vi "PH_Timing.destructor.vi"(0 "i ref in":refnum<vi>, 5 "error in(no error)":errorcluster) -> (19 "error out":errorcluster)   [LabVIEW 2014, in "PH_Timing.lvlib"]
doc: "This is the destructor of a class.\n\nLicense Agreement for this software:\n\nCopyright (C)\nGesellschaft für Schwerionenforschung, GSI\nPlanckstr. 1\n64291 Darmstadt\nGermany\n\nContact: D.Beck@gsi.de \n\nThis program is free software; you can redistribute it and/or modify it under the terms of the \nGNU General Public License as published by the Free Software Foundation; either version 2 of \nthe license, or (at your option) any later version.\n\nThis program is distributed in the hope that it will be useful, but WITHOUT ANY WARRANTY; \nwithout even the implied warranty of MERCHANTABILITY or FITNESS FOR A PARTICULAR PURPOSE. See the GNU General License for more details (http://www.gnu.org).\n\nGesellschaft für Schwerionenforschung, GSI\nPlanckstr. 1, 64291 Darmstadt, Germany\nFor all questions and ideas contact: M.Richter@gsi.de, H.Brand@gsi.de or D.Beck@gsi.de.\nLast update: 16-JUN-2004"
uses:
  PH_Timing.lvlib
  lib.lib/DimLVEvent/LVDimInterface/LVDimInterface.lvlib
  PH_Switch/PH_Switch.lvlib
  CSDigitalIO/BNC555/BNC555.lvlib
  CSDigitalIO/SRDG535/SRDG535.lvlib
  PH_SRDG645/PH_SRDG645.lvlib
  PH_Common/PH_Common.lvlib
  PH_StatusHandler/PH_StatusHandler.lvlib
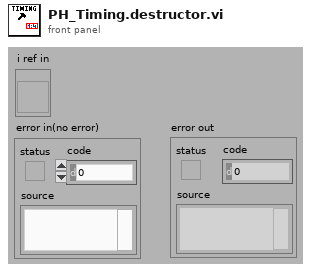
[diagram p1: front panel]
types:
  T1 = typedef "PH_Timing.lvlib/PH_Timing.i attribute.ctl" = cluster{"Sequencer":cluster{"linked?":bool, "Proc State":string, "Ref State":refnum<vi>}, "Gate Generator":cluster{"GD":cluster{"Device Status":T2, "linked?":bool}, "Settings":T3, "GUI Ref":refnum<vi>}, "Interlock Bypass":cluster{"Instancename":string, "Switch linked?":bool, "Device Status":T2, "Ref Status":refnum<vi>}, "Roughtuner":cluster{"Settings":T4, "GUI Ref":refnum<vi>, "GD":cluster{"Device Status":T2, "linked?":bool}}, "0,5Hz Gater":cluster{"Settings":T5, "GUI Ref":refnum<vi>, "GD":cluster{"Device Status":T2, "linked?":bool}}, "Slow Trigger":cluster{"Settings":T6, "GUI Ref":refnum<vi>, "Service ID Delay":i32, "Service ID Ext Trig":i32, "Wanted Settings":T6}, "Timing Mode":cluster{"Mode":T7, "GUI Ref":refnum<vi>, "Service ID T2":i32, "Service ID Mode":i32, "Wanted Mode":T7}, "ns Generator":cluster{"Settings":T8, "ns Generator Settings":refnum<vi>, "GD":cluster{"Device Status":T2, "linked?":bool}}, "Phase FEs":cluster{"Settings":T11, "GUI Ref":refnum<vi>, "Service ID Phase":i32, "Wanted Settings":T11}, "GD GUI Refs":refnum<vi>[], "Heads":T12[], "GUI Ref Delete":refnum<vi>}
  T2 = typedef "PH_StatusHandler.lvlib/PH_StatusHandler.Status.ctl" = i16
  T3 = typedef "PH_Timing.lvlib/PH_Timing.GateGen.ctl" = cluster{"Instance":string, "Channel Gate":i32, "Channel T2":i32, "Width Gate":dbl, "Width T2":dbl, "Delay Gate":dbl, "Delay T2":dbl, "Gate activ":bool, "T2 activ":bool, "System Mode":enum16{"Normal", "Single", "Burst", "Duty Cycle"}}
  T4 = typedef "PH_Timing.lvlib/PH_Timing.Roughtuner.ctl" = cluster{"Instance":string, "Phase PHELIX / UNILAC":cluster{"Channel":u16, "relative to":u16, "Delay [ms]":dbl}, "Pulse Length":cluster{"Channel":u16, "relative to":u16, "Delay [ms]":dbl}, "Trigger":cluster{"externally?":bool, "Rate [Hz]":dbl}}
  T5 = typedef "PH_Timing.lvlib/PH_Timing.0.5HzGater.ctl" = cluster{"Instance":string, "Channel ns FE Delay":i32, "Channel 0.5Hz":i32, "Width ns FE Delay":dbl, "Width 0.5Hz":dbl, "Delay ns FE Delay":dbl, "Delay 0.5Hz":dbl, "ns FE Delay active":bool, "0.5Hz activ":bool, "ns FE Delay inverted":bool, "0.5Hz inverted":bool}
  T6 = typedef "PH_Timing.lvlib/PH_Timing.Slow Trigger Settings.ctl" = cluster{"Delay":dbl, "externally triggered?":bool}
  T7 = typedef "PH_Timing.lvlib/PH_Timing.Timing Mode.ctl" = cluster{"T2":i16, "Modeselector":enum32{"10 Hz", "0.5 Hz", "Shot"}}
  T8 = typedef "PH_Timing.lvlib/PH_Timing.ns Generator.ctl" = cluster{"Instance":string, "Phase fs / ns FE":cluster{"Channel":T9, "Settings":T10}}
  T9 = typedef "Stanford Research DG645 - Driver.lvlib/Channel.ctl" = i32
  T10 = typedef "PH_SRDG645.lvlib/PH_SRDG645.Channel Settings.ctl" = cluster{"Delay [s]":dbl, "relative to":i32}
  T11 = typedef "PH_Timing.lvlib/PH_Timing.Phase FEs.ctl" = cluster{"Phase":dbl}
  T12 = typedef "PH_Timing.lvlib/PH_Timing.PU Data.ctl" = cluster{"linked?":bool, "Data":T13, "GD":cluster{"Device Status":T2, "linked?":bool}, "GUI Ref":refnum<vi>, "PU":T14}
  T13 = typedef "PH_Timing.lvlib/PH_Timing.PU Info.ctl" = cluster{"Act CH?":bool, "GD":string, "CH":i32, "Delay":dbl, "active":bool, "in Use?":bool}
  T14 = typedef "PH_PP_Common.lvlib/PH_PP_Common.PUs.ctl" = enum16{"no Info", "PA-19mm-1", "PA-19mm-2", "PA-45mm-PILC", "PA-45mm-MAIN", "MA-PU-1", "MA-PU-2", "MA-PU-3", "MA-PU-4", "MA-PU-5", "MA-PU-6", "MA-FR", "MA-PILC", "PA-45mm-DP"}
  T15 = enum16{"SetAttribute", "GetAttribute", "CreateAttribute", "DestroyAttribute", "DestroyAllAtributes"}
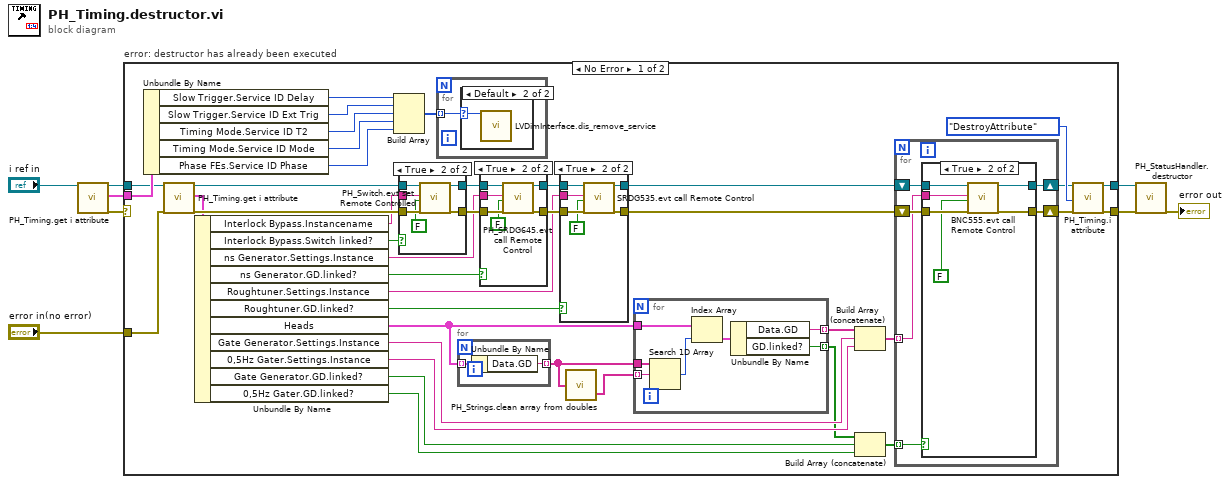
[diagram p0: block diagram]
diagram:
  n1 = call "PH_Timing.get i attribute.vi"("i ref in"="i ref in") -> ("i ref out"=w5:refnum<vi>, "i attribute"=w4:T1, "error out"=w6:errorcluster)  [unwired: 16 in]
  n2 = case "error: destructor has already been executed" shown="No Error" w6 {
    tunnel: "error in(no error)" -> [w41 w98]
    tunnel: w5 -> [w38 w99]
    tunnel: [w47 w99] -> w2
    tunnel: [w46 w98] -> w3
    tunnel: w4 -> [w45 _]
    frame No Error {
      n3 = Unbundle By Name(w45) -> ("Slow Trigger.Service ID Delay"=w36:i32, "Slow Trigger.Service ID Ext Trig"=w35:i32, "Timing Mode.Service ID T2"=w34:i32, "Timing Mode.Service ID Mode"=w33:i32, "Phase FEs.Service ID Phase"=w32:i32)
      n4 = call "PH_Timing.get i attribute.vi"("i ref in"=w38, "error in (no error)"=w41) -> ("i ref out"=w44:refnum<vi>, "i attribute"=w42:T1, "error out"=w43:errorcluster)  [unwired: 15 in]
      n5 = Unbundle By Name(w42) -> ("Interlock Bypass.Instancename"=w31:string, "Interlock Bypass.Switch linked?"=w30:bool, "ns Generator.Settings.Instance"=w26:string, "ns Generator.GD.linked?"=w29:bool, "Roughtuner.Settings.Instance"=w21:string, "Roughtuner.GD.linked?"=w20:bool, "Heads"=w9:T12[], "Gate Generator.Settings.Instance"=w16:string, "0,5Hz Gater.Settings.Instance"=w15:string, "Gate Generator.GD.linked?"=w12:bool, "0,5Hz Gater.GD.linked?"=w13:bool)
      n6 = Build Array(w36, w35, w34, w33, w32) -> (w37:i32[])
      n7 = case shown="True" w30 {
        tunnel: [w75 w81] -> w28
        tunnel: [w74 w80] -> w27
        tunnel: w44 -> [w75 w79]
        tunnel: w43 -> [w74 w78]
        tunnel: w31 -> [_ w77]
        frame False {
        }
        frame True {
          n8 = call "PH_Switch.evt set Remote Controlled.vi"("i ref in"=w79, "Instance"=w77, "Remote Controlled"=FALSE, "error in (no error)"=w78) -> ("i ref out"=w81:refnum<vi>, "error out"=w80:errorcluster)  [unwired: 14 in]
        }
      }
      n9 = for {
        tunnel: w37 -> [w82] mode=indexing
        n10 = case shown="Default" w82 {
          selector: w82 -> [_ w83]
          frame -1 {
          }
          frame Default {
            n11 = call "LVDimInterface.dis_remove_service.vi"("my_serviceID"=w83) -> ()  [unwired: 18 in, 1 out]
          }
        }
      }
      n12 = for {
        tunnel: w9 -> [w57] mode=indexing
        tunnel: [w56] -> w19 mode=indexing
        n13 = Unbundle By Name(w57) -> ("Data.GD"=w56:string)
      }
      n14 = case shown="True" w29 {
        tunnel: w28 -> [w67 w73]
        tunnel: [w67 w72] -> w25
        tunnel: w27 -> [w66 w71]
        tunnel: [w66 w70] -> w23
        tunnel: w26 -> [_ w69]
        frame False {
        }
        frame True {
          n15 = call "PH_SRDG645.evt call Remote Control.vi"("i ref in"=w73, "Generator Instance"=w69, "Remote controlled?"=FALSE, "error in (no error)"=w71) -> ("i ref out"=w72:refnum<vi>, "error out"=w70:errorcluster)  [unwired: 14 in]
        }
      }
      n16 = case shown="True" w20 {
        tunnel: w25 -> [w59 w65]
        tunnel: [w59 w64] -> w24
        tunnel: w23 -> [w58 w63]
        tunnel: [w58 w62] -> w22
        tunnel: w21 -> [_ w60]
        frame False {
        }
        frame True {
          n17 = call "SRDG535.evt call Remote Control.vi"("i ref in"=w65, "Generator Instance"=w60, "Remote controlled?"=FALSE, "error in (no error)"=w63) -> ("i ref out"=w64:refnum<vi>, "error out"=w62:errorcluster)  [unwired: 14 in]
        }
      }
      n18 = call "PH_Strings.clean array from doubles.vi"("Array Input"=w19) -> ("Cleaned Array Output"=w18:string[])  [unwired: 1 out]
      n19 = for {
        tunnel: w19 -> [w55]
        tunnel: w18 -> [w54] mode=indexing
        tunnel: w9 -> [w53]
        tunnel: [w50] -> w17 mode=indexing
        tunnel: [w49] -> w11 mode=indexing
        n20 = Search 1D Array(1D array=w55, element=w54) -> (index of element=w52:i32)  [unwired: 1 in]
        n21 = Index Array(array=w53, index=w52) -> (element=w51:T12)
        n22 = Unbundle By Name(w51) -> ("Data.GD"=w50:string, "GD.linked?"=w49:bool)
      }
      n23 = Build Array (concatenate)(w17, w16, w15) -> (w14:string[])
      n24 = Build Array (concatenate)(w11, w12, w13) -> (w10:bool[])
      n25 = for {
        shift-right: [w88] -> w40
        shift-left: w24 -> [w89]
        shift-right: [w86] -> w39
        shift-left: w22 -> [w87]
        tunnel: w14 -> [w85] mode=indexing
        tunnel: w10 -> [w84] mode=indexing
        n26 = case shown="True" w84 {
          tunnel: w89 -> [w91 w97]
          tunnel: [w91 w96] -> w88
          tunnel: w87 -> [w90 w95]
          tunnel: [w90 w94] -> w86
          tunnel: w85 -> [_ w92]
          frame False {
          }
          frame True {
            n27 = call "BNC555.evt call Remote Control.vi"("i ref in"=w97, "Generator Instance"=w92, "Remote controlled?"=FALSE, "error in (no error)"=w95) -> ("i ref out"=w96:refnum<vi>, "error out"=w94:errorcluster)  [unwired: 14 in]
          }
        }
      }
      n28 = call "PH_Timing.i attribute.vi"("VI Refnum"=w40, "Action"=T15."DestroyAttribute", "error in (no error)"=w39) -> ("VI Refnum out"=w47:refnum<vi>, "error out"=w46:errorcluster)  [unwired: 14 in, 1 out]
    }
    frame Error {
    }
  }
  n29 = call "PH_StatusHandler.destructor.vi"("i ref in"=w2, "error in(no error)"=w3) -> ("error out"=→"error out":errorcluster)  [unwired: 17 in]
